vi "Basic Security Configuration From Path.vi"(1 "Current Path":path) -> (0 "Basic Security Settings":T1)   [LabVIEW 2012]
doc: "Creates a basic security configuration."
uses:
  RTI/GIT_HEAD/connextdds/lvdds.1.0/srcLV/lvdds.1.0_package/Types/RTI DDS Basic Security Settings.ctl
  RTI/GIT_HEAD/connextdds/lvdds.1.0/srcLV/lvdds.1.0_package/Library/LVDDS_library.lvlib
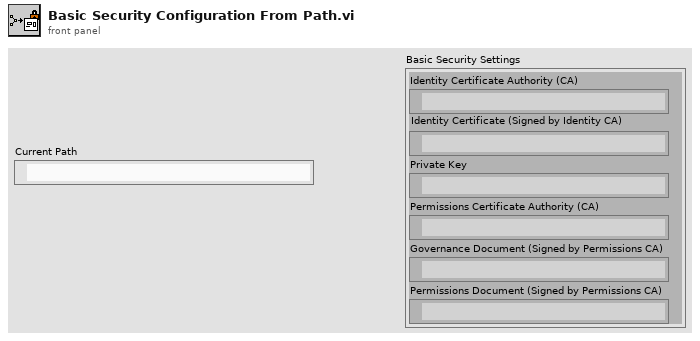
[diagram p1: front panel]
types:
  T1 = typedef "LVDDS_library.lvlib/RTI DDS Basic Security Settings.ctl" = cluster{"Identity Certificate Authority (CA)":path, "Identity Certificate (Signed by Identity CA)":path, "Private Key":path, "Permissions Certificate Authority (CA)":path, "Governance Document (Signed by Permissions CA)":path, "Permissions Document (Signed by Permissions CA)":path}
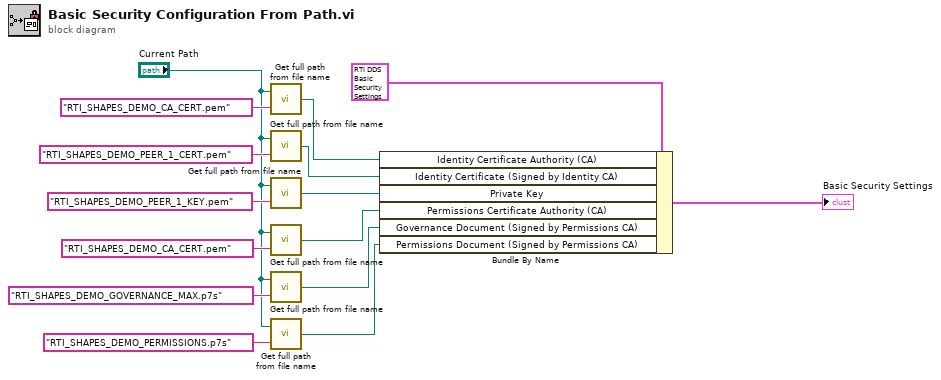
[diagram p0: block diagram]
diagram:
  n1 = call "Get full path from file name.vi"("File Name"="RTI_SHAPES_DEMO_CA_CERT.pem" ("name or relative path"), "Current Path"="Current Path") -> ("Full Path"=w8:path)
  n2 = call "Get full path from file name.vi"("File Name"="RTI_SHAPES_DEMO_PEER_1_CERT.pem" ("name or relative path"), "Current Path"="Current Path") -> ("Full Path"=w7:path)
  n3 = call "Get full path from file name.vi"("File Name"="RTI_SHAPES_DEMO_PEER_1_KEY.pem" ("name or relative path"), "Current Path"="Current Path") -> ("Full Path"=w1:path)
  n4 = call "Get full path from file name.vi"("File Name"="RTI_SHAPES_DEMO_CA_CERT.pem" ("name or relative path"), "Current Path"="Current Path") -> ("Full Path"=w6:path)
  n5 = call "Get full path from file name.vi"("File Name"="RTI_SHAPES_DEMO_GOVERNANCE_MAX.p7s" ("name or relative path"), "Current Path"="Current Path") -> ("Full Path"=w5:path)
  n6 = call "Get full path from file name.vi"("File Name"="RTI_SHAPES_DEMO_PERMISSIONS.p7s" ("name or relative path"), "Current Path"="Current Path") -> ("Full Path"=w4:path)
  n7 = Bundle By Name(cluster=T1 {"Identity Certificate Authority (CA)"=path "", "Identity Certificate (Signed by Identity CA)"=path "", "Private Key"=path "", "Permissions Certificate Authority (CA)"=path "", "Governance Document (Signed by Permissions CA)"=path "", "Permissions Document (Signed by Permissions CA)"=path ""} ("Basic Security Settings 2"), "Identity Certificate Authority (CA)"=w8, "Identity Certificate (Signed by Identity CA)"=w7, "Private Key"=w1, "Permissions Certificate Authority (CA)"=w6, "Governance Document (Signed by Permissions CA)"=w5, "Permissions Document (Signed by Permissions CA)"=w4) -> (→"Basic Security Settings":T1)
